vi "self-resetting-iter.vi"(11 "zup-N":i16) -> (0 "Numeric":i16, 3 "Boolean":bool)   [LabVIEW 2015, in "libimaging-cs.lvlib"]
uses:
  libimaging-cs.lvlib
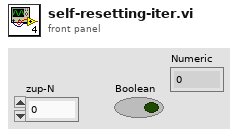
[diagram p1: front panel]
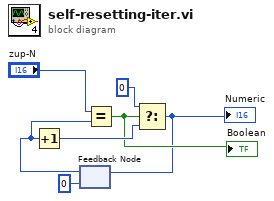
[diagram p0: block diagram]
diagram:
  n1 = feedback #1(i16 0) -> (w5:i16)
  n2 = Increment(x=w5) -> (x+1=w6:i16)
  n3 = Equal?(x="zup-N", y=w5) -> (x = y?=w2:bool)
  "Boolean" <- w2
  n4 = Select(t=i16 0, s=w2, f=w6) -> (s? t:f=w1:i16)
  "Numeric" <- w1
  n5 = feedback-in #1(w1) -> ()
